vi "ShoulderRead.vi"(0 "error in":errorcluster, 2 "Side":T1=enum."right", 3 "node":string) -> (1 "error out":errorcluster, 4 "Pushed":bool)   [LabVIEW 2013]
doc: "This VI gets the status of the Navigator Buttons"
uses:
  ROS/Code/SubVIs/BaxterSide.ctl
  ROS/parsing/primitives/subs/parse_i8_scalar.vi
panel:
  out "Reply":string
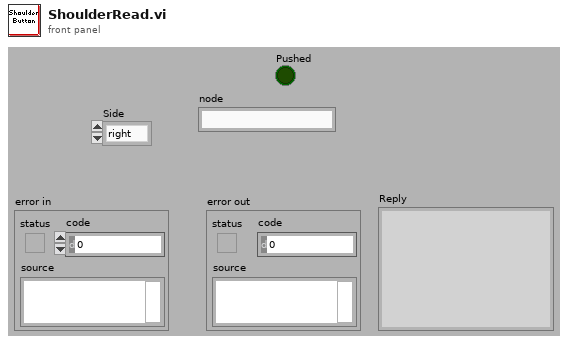
[diagram p1: front panel]
types:
  T1 = typedef "BaxterSide.ctl" = enum16{"left", "right"}
  T2 = typedef "_ROSControl.ctl" = cluster{"topic port":u16, "Node":string, "topic":string, "type":string, "node port":u32, "error ":errorcluster, "Direction":T3, "APIs":string[]}
  T3 = typedef "_ROSDirection.ctl" = enum16{"Node", "Publisher", "Subscriber", "Service Client"}
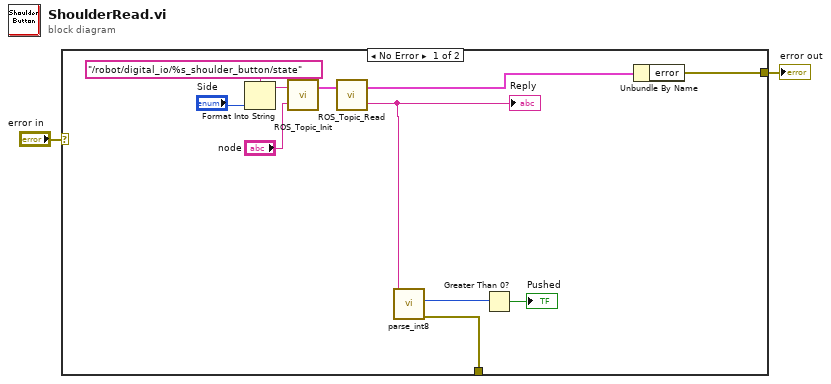
[diagram p0: block diagram]
diagram:
  n1 = case shown="No Error" "error in" {
    selector: "error in" -> [_ w14]
    tunnel: [w13 w14] -> w2
    tunnel: [w5 _] -> _
    frame No Error {
      n2 = Format Into String(format string="/robot/digital_io/%s_shoulder_button/state" ("topic"), "Side") -> (resulting string=w8:string)  [unwired: 2 in, 1 out]
      n3 = call "ROS_Topic_Init.vi"("node"="node", "topic"=w8) -> ("ROS out"=w11:T2)  [unwired: 1 in]
      n4 = call "ROS_Topic_Read.vi"("ROS in"=w11) -> ("Reply"=w7:string, "ROS out"=w10:T2)  [unwired: 1 in]
      "Reply" <- w7
      n5 = call-poly "parse_int8.vi"("msg in"=w7) -> ("error out"=w5:errorcluster, "number"=w4:i8)  [unwired: 4 in, 1 out]
      n6 = Greater Than 0?(x=w4) -> (x > 0?=→"Pushed":bool)
      n7 = Unbundle By Name(w10) -> ("error"=w13:errorcluster)
    }
    frame Error {
    }
  }
  "error out" <- w2
